vi "DO-NOT-USE_getDelay.vi"(8 "error in (no error)":errorcluster, 11 "Instrument.Delay in":refnum<class "Instrument.Aerotech.lvclass">) -> (0 "error out":errorcluster, 2 "Delay (ps)":dbl, 3 "Instrument.Delay out":refnum<class "Instrument.Aerotech.lvclass">, 4 "Finished?":bool)   [LabVIEW 2019, in "Instrument.Aerotech.lvclass"]
uses:
  Instrument.Aerotech.lvclass
  Instrument.Aerotech.lvclass/Instrument.Aerotech.ctl
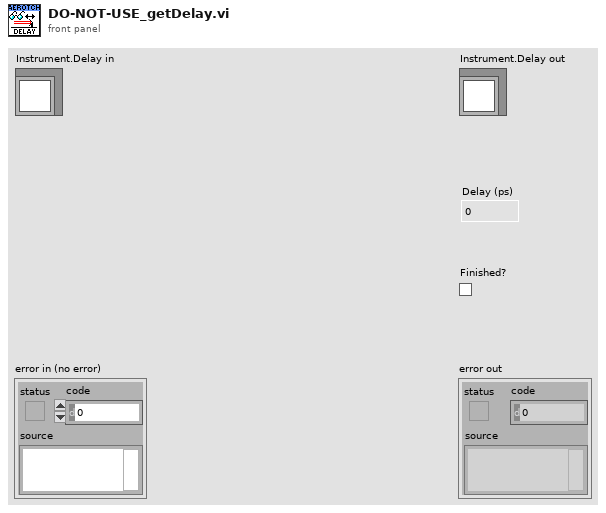
[diagram p1: front panel]
types:
  T1 = typedef "ControllerDiagPacket.ctl" = cluster{"Count":i32, "Packet Time":i64, "Axes":T2[], "error":errorcluster}
  T2 = typedef "AxisDiagPacket.ctl" = cluster{"Axis Name":string, "Acceleration Command":dbl, "Amplifier Temperature":sgl, "Analog Input 0":dbl, "Analog Input 1":dbl, "Analog Output 0":dbl, "Analog Output 1":dbl, "Axis Fault (num)":i32, "Axis Fault (str)":string, "Axis Fault (bits)":cluster{"AmplifierFault":bool, "AmplifierTemperatureFault":bool, "CcwEndOfTravelLimitFault":bool, "CcwSoftwareLimitFault":bool, "CommunicationLostFault":bool, "CwEndOfTravelLimitFault":bool, "CwSoftwareLimitFault":bool, "EmergencyStopFault":bool, "EncoderFault":bool, "ExternalFault":bool, "FeedbackScalingFault":bool, "HallSensorFault":bool, "MarkerSearchFault":bool, "MaxVelocityCommandFault":bool, "MotorTemperatureFault":bool, "None":bool, "OverCurrentFault":bool, "PositionErrorFault":bool, "PositionFeedbackFault":bool, "PowerSupplyFault":bool, "VelocityErrorFault":bool, "VelocityFeedbackFault":bool, "VoltageClampFault":bool}, "Axis Status (num)":i32, "Axis Status (str)":string, "Axis Status (bits)":cluster{"AccelerationPhase":bool, "AutofocusActive":bool, "BrakeOutput":bool, "CalibrationActive":bool, "CalibrationEnabled":bool, "CcwEndOfTravelLimitInput":bool, "CommandShapingFilterDone":bool, "CosineEncoderError":bool, "CurrentClamp":bool, "CwEndOfTravelLimitInput":bool, "DecelerationPhase":bool, "EmergencyStopInput":bool, "Enabled":bool, "GantryMasterActive":bool, "GantryModeActive":bool, "HallAInput":bool, "HallBInput":bool, "HallCInput":bool, "Homed":bool, "HomeLimitInput":bool, "Homing":bool, "InPosition":bool, "InPosition2":bool, "JoystickControl":bool, "MarkerInput":bool, "MasterMotionSuppressed":bool, "MasterSlaveControl":bool, "MotionIsCw":bool, "MoveActive":bool, "None":bool, "PositionCaptureActive":bool, "ServoControl":bool, "SineEncoderError":bool}, "Current Command":sgl, "Current Error":sgl, "Current Feedback":sgl, "Digital Input 0":i32, "Digital Input 1":i32, "Digital Input 2":i32, "Digital Output 0":i32, "Digital Output 1":i32, "Digital Output 2":i32, "Position Feedback Auxiliary":dbl, "Position Command":dbl, "Position Error":dbl, "Position Feedback":dbl, "Program Position Command":dbl, "Program Position Error":dbl, "Program Position Feedback":dbl, "Velocity Command":dbl, "Velocity Error":dbl, "Velocity Feedback":dbl}
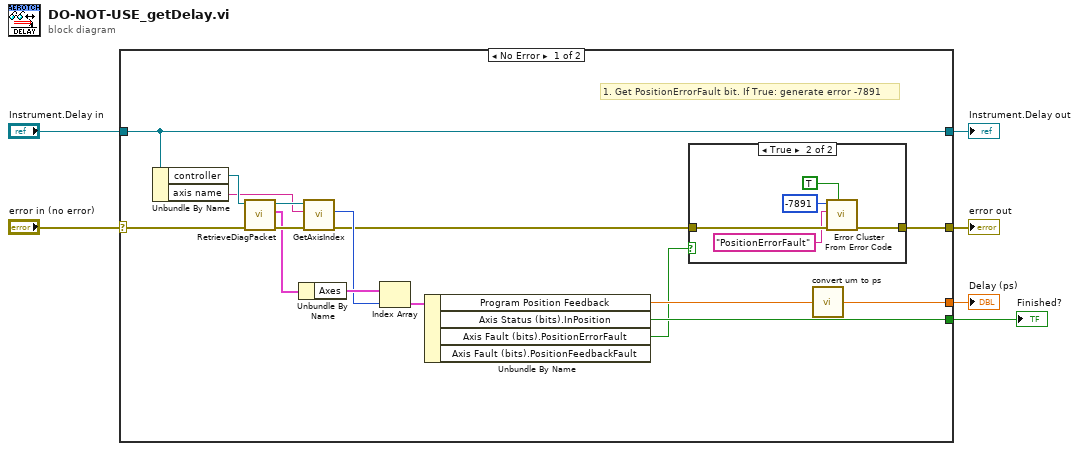
[diagram p0: block diagram]
diagram:
  n1 = case shown="No Error" "error in (no error)" {
    selector: "error in (no error)" -> [w13 w30]
    tunnel: [w9 w30] -> w6
    tunnel: [w11 _] -> w5
    tunnel: [w16 _] -> w4
    tunnel: "Instrument.Delay in" -> [w8 w29]
    tunnel: [w8 w29] -> w1
    frame No Error {
      # "1. Get PositionErrorFault bit. If True: generate error -7891"
      n2 = Unbundle By Name(w8) -> ("controller"=w15:refnum<k24>, "axis name"=w14:string)
      n3 = call "RetrieveDiagPacket.vi"("error in (no error)"=w13, "Controller In"=w15) -> ("error out"=w21:errorcluster, "ControllerDiagPacket"=w20:T1, "Controller Out"=w22:refnum<k24>)  [unwired: 7 in]
      n4 = Unbundle By Name(w20) -> ("Axes"=w19:T2[])
      n5 = call "GetAxisIndex.vi"("error in (no error)"=w21, "axis name"=w14, "controller in"=w22) -> ("error out"=w10:errorcluster, "axis index"=w18:i32)  [unwired: 6 in, 1 out]
      n6 = Index Array(array=w19, index=w18) -> (element=w17:T2)
      n7 = Unbundle By Name(w17) -> ("Program Position Feedback"=w12:dbl, "Axis Status (bits).InPosition"=w16:bool, "Axis Fault (bits).PositionErrorFault"=w7:bool)  [unwired: 1 out]
      n8 = case shown="True" w7 {
        tunnel: w10 -> [w23 w28]
        tunnel: [w23 w27] -> w9
        frame False {
        }
        frame True {
          n9 = call <vilib>:"Error Cluster From Error Code.vi"("show call chain? (False)"=TRUE, "error in (no error)"=w28, "error message (\"\")"="PositionErrorFault" ("error message (\"\")"), "error code (0)"=-7891) -> ("error out"=w27:errorcluster)  [unwired: 5 in]
        }
      }
      n10 = call "convert um to ps.vi"("Position (um)"=w12) -> ("Delay (ps)"=w11:dbl)
    }
    frame Error {
    }
  }
  "error out" <- w6
  "Instrument.Delay out" <- w1
  "Delay (ps)" <- w5
  "Finished?" <- w4
